vi "Create Object.vi"(6 "instanceId":i32, 8 "error in (no error)":errorcluster, 9 "attributes":cluster{"name":string, "type":string}[](array[cluster]), 10 "name":string, 11 "Item Ref in":T1 format="%.0x") -> (0 "error out":errorcluster, 3 "Item Ref out":T1 format="%.0x")   [LabVIEW 2019, in "HLA Custom Device System Explorer.lvlib"]
uses:
  HLA Custom Device System Explorer.lvlib
  <vilib>/NI VeriStand/Custom Device API/Custom Device Item Ref.ctl
  Shared/Constants.vi
  <vilib>/NI VeriStand/Custom Device API/Set Item Property (I32).vi
  <vilib>/NI VeriStand/Custom Device API/Custom Device API.lvlib
  Shared/HLA Custom Device Shared.lvlib
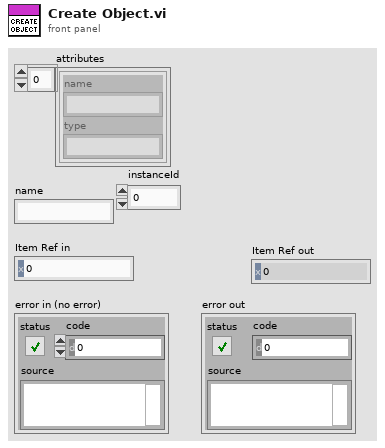
[diagram p1: front panel]
types:
  T1 = typedef "Custom Device API.lvlib/Custom Device Item Ref.ctl" = u64
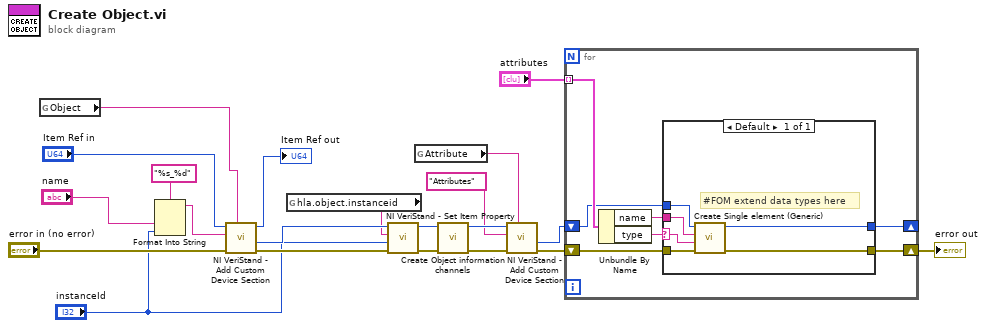
[diagram p0: block diagram]
diagram:
  n1 = global read "Constants.vi" "Object"() -> (w15:string)
  n2 = Format Into String(format string="%s_%d", "name", "instanceId") -> (resulting string=w1:string)  [unwired: 2 in, 1 out]
  n3 = call <vilib>:"NI VeriStand - Add Custom Device Section.vi"("GUID (Default Section)"=w15, "error in (no error)"="error in (no error)", "Section Name"=w1, "Parent Ref in"="Item Ref in") -> ("error out"=w6:errorcluster, "Section Ptr"=w7:T1, "Parent Ref out"=→"Item Ref out":T1)  [unwired: 4 in, 1 out]
  n4 = global read "Constants.vi" "hla.object.instanceid"() -> (w5:string)
  n5 = call-poly <vilib>:"NI VeriStand - Set Item Property.vi"("error in (no error)"=w6, "Value"="instanceId", "Property Name"=w5, "Item Ref in"=w7) -> ("error out"=w8:errorcluster, "Item Ref out"=w9:T1)  [unwired: 5 in, 1 out]
  n6 = global read "Constants.vi" "Attribute"() -> (w21:string)
  n7 = call "Create Object information channels.vi"("error in"=w8, "Item Ref in"=w9) -> ("error out"=w17:errorcluster, "Item Ref out"=w18:T1)  [unwired: 8 in]
  n8 = call <vilib>:"NI VeriStand - Add Custom Device Section.vi"("GUID (Default Section)"=w21, "error in (no error)"=w17, "Section Name"="Attributes", "Parent Ref in"=w18) -> ("error out"=w20:errorcluster, "Section Ptr"=w19:T1)  [unwired: 4 in, 2 out]
  n9 = for {
    shift-right: [w22] -> w13
    shift-left: w20 -> [w26]
    tunnel: "attributes" -> [w28] mode=indexing
    shift-right: [w23] -> _
    shift-left: w19 -> [w25]
    n10 = Unbundle By Name(w28) -> ("name"=w24:string, "type"=w27:string)
    n11 = case shown="Default" w27 {
      selector: w27 -> [w31]
      tunnel: w26 -> [w33]
      tunnel: w25 -> [w34]
      tunnel: w24 -> [w32]
      tunnel: [w30] -> w23
      tunnel: [w29] -> w22
      frame Default {
        # "#FOM extend data types here"
        n12 = call "Create Single element (Generic).vi"("error in"=w33, "type"=w31, "name"=w32, "Item Ref in"=w34) -> ("error out"=w29:errorcluster, "Item Ref out"=w30:T1)  [unwired: 6 in]
      }
    }
  }
  "error out" <- w13
